vi "StripPath_ListFolderContents.vi"(8 "error in (no error)":errorcluster, 11 "Config":T1) -> (0 "error out":errorcluster, 3 "filenames":string[](array[string]))   [LabVIEW 2014]
doc: "This VI takes a file path, strips the filename and then lists the parent folder's contents in a string array."
uses:
  Settings/Settings.ctl
  Acquisition/Hardware Configuration.ctl
  Logging/Logging Configuration.ctl
  Acquisition/Acquisition.lvlib
  Settings/Settings.lvlib
  Logging/Logging.lvlib
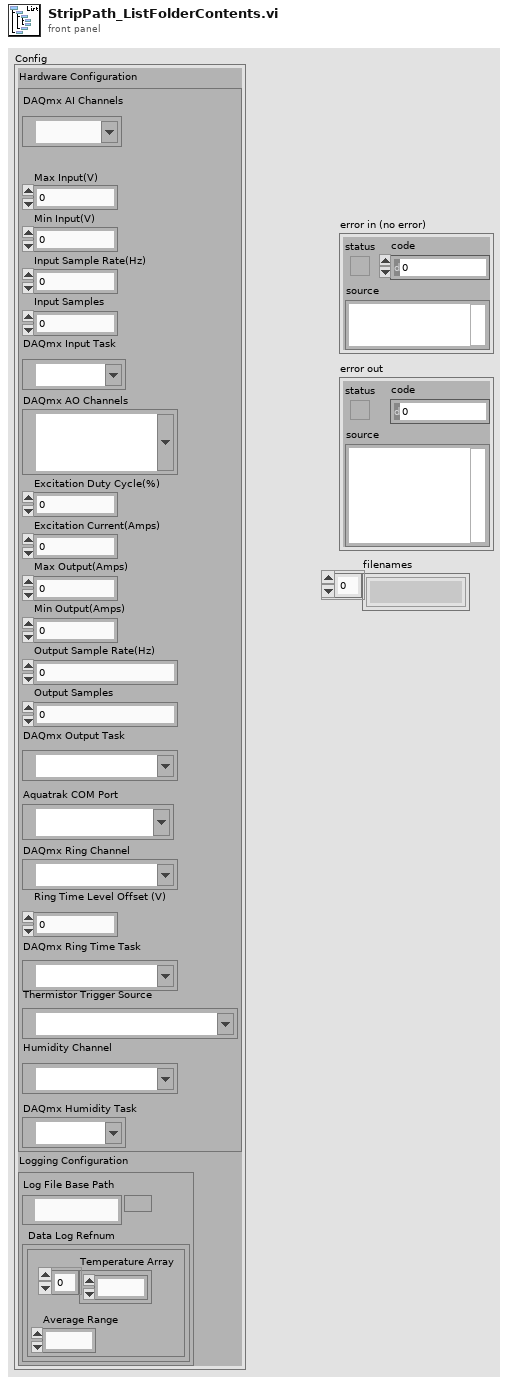
[diagram p1: front panel]
types:
  T1 = typedef "Settings.lvlib/Settings.ctl" = cluster{"Hardware Configuration":T2, "Logging Configuration":T3}
  T2 = typedef "Acquisition.lvlib/Hardware Configuration.ctl" = cluster{"DAQmx AI Channels":tag, "Max Input(V)":dbl, "Min Input(V)":dbl, "Input Sample Rate(Hz)":dbl, "Input Samples":dbl, "DAQmx Input Task":refnum<k21>, "DAQmx AO Channels":tag, "Excitation Duty Cycle(%)":dbl, "Excitation Current(Amps)":dbl, "Max Output(Amps)":dbl, "Min Output(Amps)":dbl, "Output Sample Rate(Hz)":dbl, "Output Samples":dbl, "DAQmx Output Task":refnum<k21>, "Aquatrak COM Port":refnum<visa-resource-name>, "DAQmx Ring Channel":tag, "Ring Time Level Offset (V)":dbl, "DAQmx Ring Time Task":refnum<k21>, "Thermistor Trigger Source":tag, "Humidity Channel":tag, "DAQmx Humidity Task":refnum<k21>}
  T3 = typedef "Logging.lvlib/Logging Configuration.ctl" = cluster{"Log File Base Path":path, "Data Log Refnum":refnum<k1>}
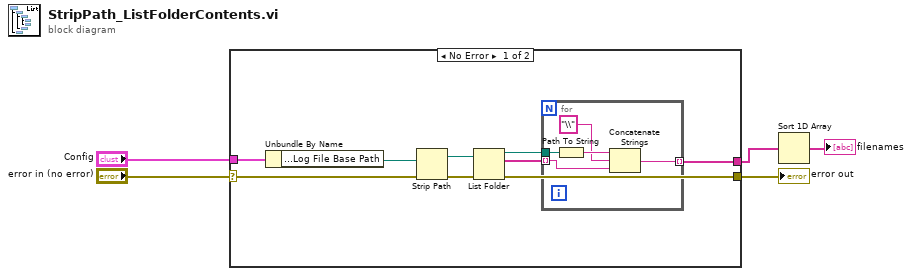
[diagram p0: block diagram]
diagram:
  n1 = case shown="No Error" "error in (no error)" {
    selector: "error in (no error)" -> [w10 w19]
    tunnel: [w9 w19] -> w5
    tunnel: "Config" -> [w12 _]
    tunnel: [w6 _] -> w2
    frame No Error {
      n2 = Unbundle By Name(w12) -> ("Logging Configuration.Log File Base Path"=w13:path)
      n3 = Strip Path(path=w13) -> (stripped path=w11:path)  [unwired: 1 out]
      n4 = List Folder(path=w11, error in=w10) -> (path out=w7:path, filenames=w8:string[], error out=w9:errorcluster)  [unwired: 2 in, 1 out]
      n5 = for {
        tunnel: w8 -> [w14] mode=indexing
        tunnel: w7 -> [w18]
        tunnel: [w16] -> w6 mode=indexing
        n6 = Path To String(path=w18) -> (string=w17:string)
        n7 = Concatenate Strings(w17, "\\" ("string"), w14) -> (w16:string)
      }
    }
    frame Error {
    }
  }
  "error out" <- w5
  n8 = Sort 1D Array(array=w2) -> (sorted array=→"filenames":string[])
